vi "Giro controlado sobre eje.vi"   [LabVIEW 2020]
uses:
  <vilib>/Rock Robotics/WPI/Utilities/WPI_GetSetVariantRefNum.vi
  2022 Robot Project TEST 1/GiroL or GiroR.vi
types:
  T1 = typedef "WPI_JoystickDevRef.ctl" = cluster{"Device":T2}
  T2 = typedef "WPI_JoystickDeviceEnum.ctl" = enum16{"USB 0", "USB 1", "USB 2", "USB 3", "USB 4", "USB 5"}
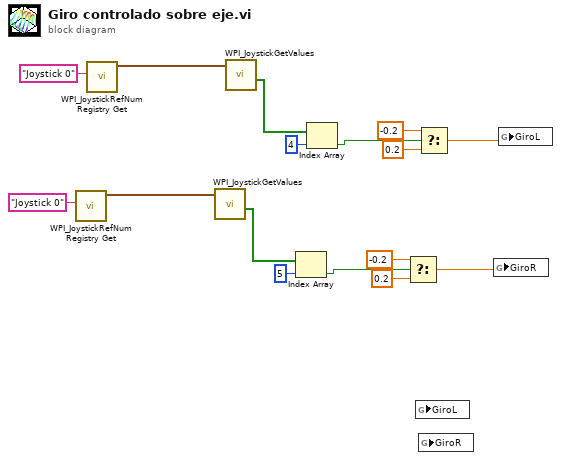
[diagram p0: block diagram]
diagram:
  n1 = call <vilib>:"WPI_JoystickRefNum Registry Get.vi"("refnum name"="Joystick 0") -> ("JoystickDevRef"=w10:T1)  [unwired: 9 in, 1 out]
  n2 = call <vilib>:"WPI_JoystickRefNum Registry Get.vi"("refnum name"="Joystick 0") -> ("JoystickDevRef"=w15:T1)  [unwired: 9 in, 1 out]
  n3 = call <vilib>:"WPI_JoystickGetValues.vi"("JoystickDevRef"=w10) -> ("Buttons"=w9:bool[])  [unwired: 6 in, 4 out]
  n4 = call <vilib>:"WPI_JoystickGetValues.vi"("JoystickDevRef"=w15) -> ("Buttons"=w14:bool[])  [unwired: 6 in, 4 out]
  n5 = Index Array(array=w9, index=5) -> (element=w7:bool)
  n6 = Index Array(array=w14, index=4) -> (element=w12:bool)
  n7 = Select(t=-0.2, s=w7, f=0.2) -> (s? t:f=w5:dbl)
  n8 = global read "GiroL or GiroR.vi" "GiroL"() -> ()  [unwired: 1 in]
  n9 = Select(t=-0.2, s=w12, f=0.2) -> (s? t:f=w6:dbl)
  n10 = global read "GiroL or GiroR.vi" "GiroR"() -> ()  [unwired: 1 in]
  n11 = global write "GiroL or GiroR.vi" "GiroR"(w5) -> ()
  n12 = global write "GiroL or GiroR.vi" "GiroL"(w6) -> ()
